vi "TangoConnect.vi"(9 "show Protocol":bool, 11 "Tango Com":refnum<visa-resource-name>) -> (0 "error out":errorcluster, 2 "success":bool, 3 "plLSID out":i32, 10 "Baud":dbl)   [LabVIEW 2018]
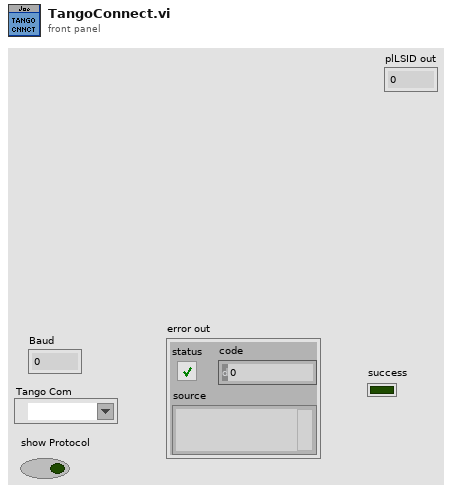
[diagram p1: front panel]
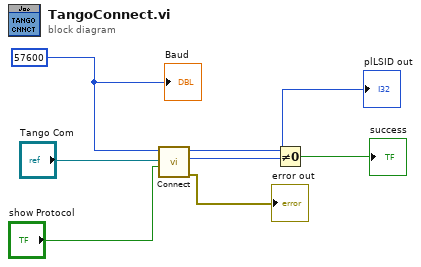
[diagram p0: block diagram]
diagram:
  w6 = 57600 ("lABaudRate")
  n1 = call "Connect.vi"("ShProt?"="show Protocol", "pcAComName"="Tango Com", "lABaudRate"=w6) -> ("error out"=→"error out":errorcluster, "function return"=w2:i32, "plLSID out"=→"plLSID out":i32)  [unwired: 5 in]
  n2 = Not Equal To 0?(x=w2) -> (x != 0?=→"success":bool)
  "Baud" <- w6
